vi "Extract Rotation.vi"(1 "Transformation matrix":T1) -> (0 "Rotation matrix":T1)   [LabVIEW 2024]
uses:
  <vilib>/Analysis/Matrix/Datatypes/RealMatrix.ctl
  <vilib>/Analysis/Matrix/NI_Matrix.lvlib
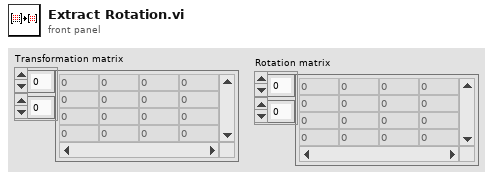
[diagram p1: front panel]
types:
  T1 = typedef "NI_Matrix.lvlib/RealMatrix.ctl" = dbl[][]
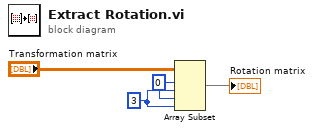
[diagram p0: block diagram]
diagram:
  w2 = 3 ("disabled index (col)")
  w3 = 0 ("index")
  n1 = Array Subset(array="Transformation matrix", index (row)=w3, length (row)=w2, index (col)=w3, length (col)=w2) -> (→"Rotation matrix":T1)
